vi "InitTrendPoint.vi"(6 "DataGroups":T1[](array[typedef]), 8 "error in (no error)":errorcluster, 9 "AssetNodeId":string, 10 "DataGroup":string, 11 "trend registrations in":variant) -> (0 "error out":errorcluster, 2 "groups":string[](array[string]), 3 "trend registrations out":variant)   [LabVIEW 2017, in "ModbusMaster.lvlib"]
uses:
  <vilib>/addons/InsightCM/Devices/Shared/Common/ModbusMaster/ModbusMaster.lvlib
  <vilib>/addons/InsightCM/MessageBus/Base/controls/R2_DataGroup.ctl
  <vilib>/addons/InsightCM/MessageBus/Base/controls/OperatingState.ctl
  <vilib>/addons/InsightCM/MessageBus/Base/controls/KeyValuePair.ctl
  <vilib>/addons/InsightCM/MessageBus/Base/controls/Trigger.ctl
  <vilib>/addons/InsightCM/MessageBus/Base/controls/Condition.ctl
  <vilib>/addons/PointValueMap/subVIs/Point_Create_double.vi
  <vilib>/addons/PointValueMap/PointValueMap.lvlib
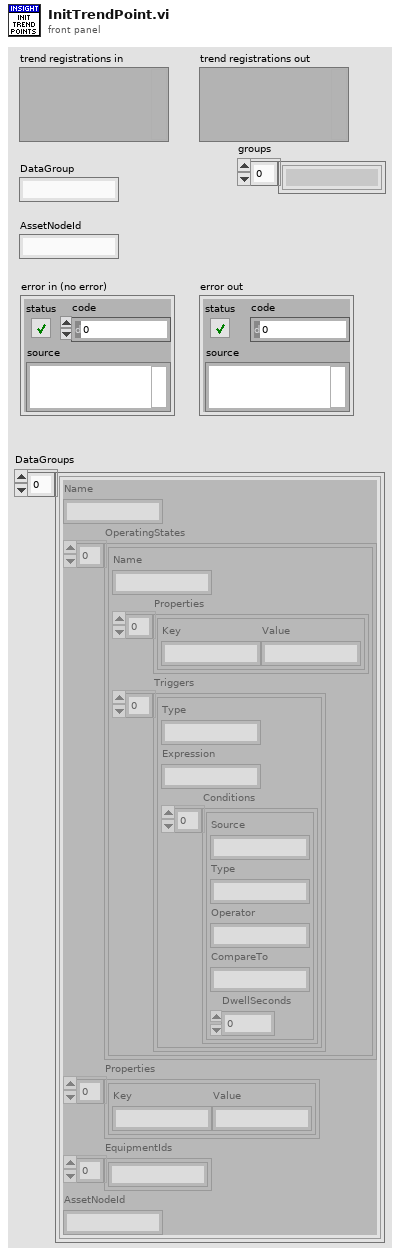
[diagram p1: front panel]
types:
  T1 = typedef "R2_DataGroup.ctl" = cluster{"Name":string, "OperatingStates":T2[], "Properties":T3[], "EquipmentIds":string[], "AssetNodeId":string}
  T2 = typedef "OperatingState.ctl" = cluster{"Name":string, "Properties":T3[], "Triggers":T4[]}
  T3 = typedef "KeyValuePair.ctl" = cluster{"Key":string, "Value":string}
  T4 = typedef "Trigger.ctl" = cluster{"Type":string, "Expression":string, "Conditions":T5[]}
  T5 = typedef "Condition.ctl" = cluster{"Source":string, "Type":string, "Operator":string, "CompareTo":string, "DwellSeconds":dbl}
  T6 = typedef "PointValueMap.lvlib/PointMap.ctl" = refnum<data-value>
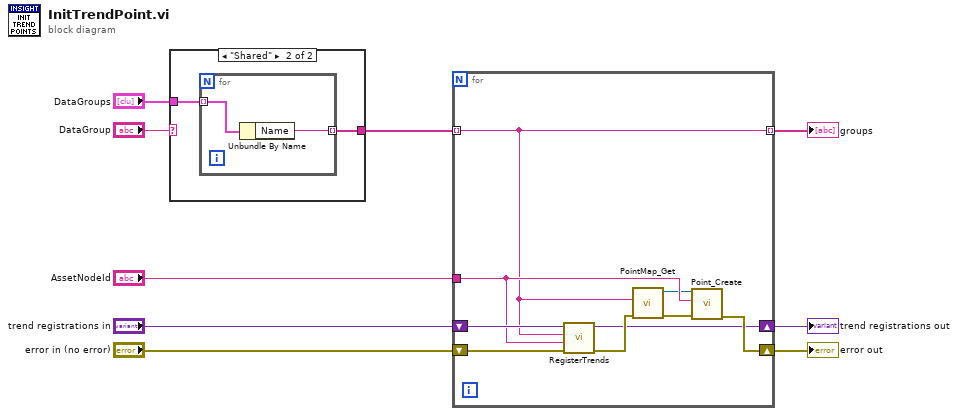
[diagram p0: block diagram]
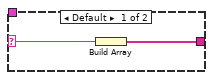
[diagram p2: hidden frame]
diagram:
  n1 = case shown="\"Shared\"" "DataGroup" {
    selector: "DataGroup" -> [w11 _]
    tunnel: [w10 w12] -> w3
    tunnel: "DataGroups" -> [_ w13]
    frame Default {
      n2 = Build Array(w11) -> (w10:string[])
    }
    frame "Shared" {
      n3 = for {
        tunnel: w13 -> [w15] mode=indexing
        tunnel: [w14] -> w12 mode=indexing
        n4 = Unbundle By Name(w15) -> ("Name"=w14:string)
      }
    }
  }
  n5 = for {
    tunnel: "AssetNodeId" -> [w19]
    shift-right: [w24] -> w9
    shift-left: "error in (no error)" -> [w22]
    shift-right: [w20] -> w6
    shift-left: "trend registrations in" -> [w21]
    tunnel: w3 -> [w16] mode=indexing
    tunnel: [w16] -> w1 mode=indexing
    n6 = call <vilib>:"RegisterTrends.vi"("error in (no error)"=w22, "asset node id"=w19, "data group"=w16, "data group map"=w21) -> ("error out"=w23:errorcluster, "data group map"=w20:variant)  [unwired: 6 in]
    n7 = call <vilib>:"PointMap_Get.vi"("error in (no error)"=w23, "Name"=w16) -> ("error out"=w17:errorcluster, "Map Out"=w18:T6)  [unwired: 7 in, 1 out]
    n8 = call-poly <vilib>:"Point_Create.vi"("Error In"=w17, "Tag"=w19, "Map"=w18) -> ("Error Out"=w24:errorcluster)  [unwired: 7 in, 1 out]
  }
  "error out" <- w9
  "trend registrations out" <- w6
  "groups" <- w1
